vi "FT10_Semi-Auto Set Power Display String.vi"(11 "Auto Set Power Cluster":T1 {"Power Level" format="%.1f"}) -> (3 "Display String":string)   [LabVIEW 2024]
doc: "Create string to send to Update Display case to show user what power level has been set."
uses:
  Controls/Control_Auto Set Power Cluster.ctl
  Controls/Control_Semi-Auto Port.ctl
  Controls/Control_Semi-Auto Mode.ctl
  Controls/Control_Semi-Auto Power Level.ctl
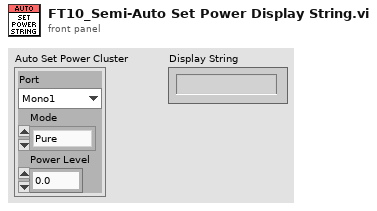
[diagram p1: front panel]
types:
  T1 = typedef "Control_Auto Set Power Cluster.ctl" = cluster{"Port":T2, "Mode":T3, "Power Level":T4}
  T2 = typedef "Control_Semi-Auto Port.ctl" = enum16{"Mono1", "Mono2", "Bipolar", "Ligasure", "Error"}
  T3 = typedef "Control_Semi-Auto Mode.ctl" = enum16{"Pure", "Blend", "Spray", "Fulgerate", "Standard", "Macro", "Precision", "Ligasure", "Error"}
  T4 = typedef "Control_Semi-Auto Power Level.ctl" = dbl
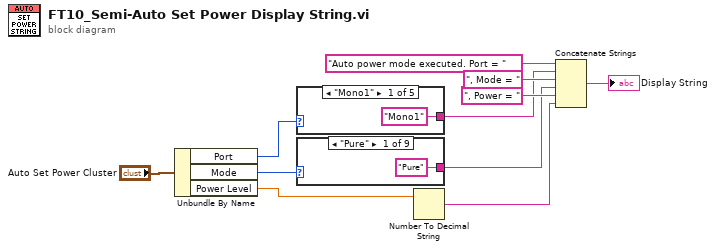
[diagram p0: block diagram]
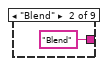
[diagram p2: hidden frame]
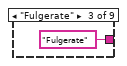
[diagram p3: hidden frame]
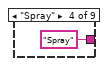
[diagram p4: hidden frame]
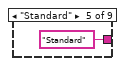
[diagram p5: hidden frame]
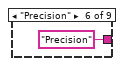
[diagram p6: hidden frame]
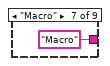
[diagram p7: hidden frame]
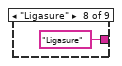
[diagram p8: hidden frame]
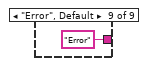
[diagram p9: hidden frame]
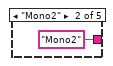
[diagram p10: hidden frame]
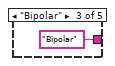
[diagram p11: hidden frame]
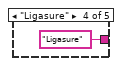
[diagram p12: hidden frame]
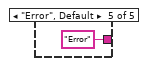
[diagram p13: hidden frame]
diagram:
  n1 = Unbundle By Name("Auto Set Power Cluster") -> ("Port"=w9:T2, "Mode"=w8:T3, "Power Level"=w11:T4)
  n2 = case shown="\"Mono1\"" w9 {
    tunnel: ["Mono1" ("Port") "Mono2" ("Port") "Bipolar" ("Port") "Ligasure" ("Port") "Error" ("Port")] -> w4
    frame "Mono1" {
    }
    frame "Mono2" {
    }
    frame "Bipolar" {
    }
    frame "Ligasure" {
    }
    frame "Error", Default {
    }
  }
  n3 = case shown="\"Pure\"" w8 {
    tunnel: ["Pure" ("Port") "Blend" ("Port") "Fulgerate" ("Port") "Spray" ("Port") "Standard" ("Port") "Precision" ("Port") "Macro" ("Port") "Ligasure" ("Port") "Error" ("Port")] -> w3
    frame "Pure" {
    }
    frame "Blend" {
    }
    frame "Fulgerate" {
    }
    frame "Spray" {
    }
    frame "Standard" {
    }
    frame "Precision" {
    }
    frame "Macro" {
    }
    frame "Ligasure" {
    }
    frame "Error", Default {
    }
  }
  n4 = Number To Decimal String(number=w11) -> (decimal integer string=w2:string)  [unwired: 1 in]
  n5 = Concatenate Strings("Auto power mode executed. Port = " ("string"), w4, ", Mode = " ("string"), w3, ", Power = " ("string"), w2) -> (→"Display String":string)
